vi "PulseParseSequence.vi"(0 "String":string) -> (1 "Step invarient?":bool, 2 "pulses cluster":T1)   [LabVIEW 2017]
panel:
  out "Camera String":string
  out "Sequences cluster":T2
  out "RF String":string
  out "Main Pulses String":string
  out "Synths String":string
  out "Pars String":string
  out "Aux Pulses String":string
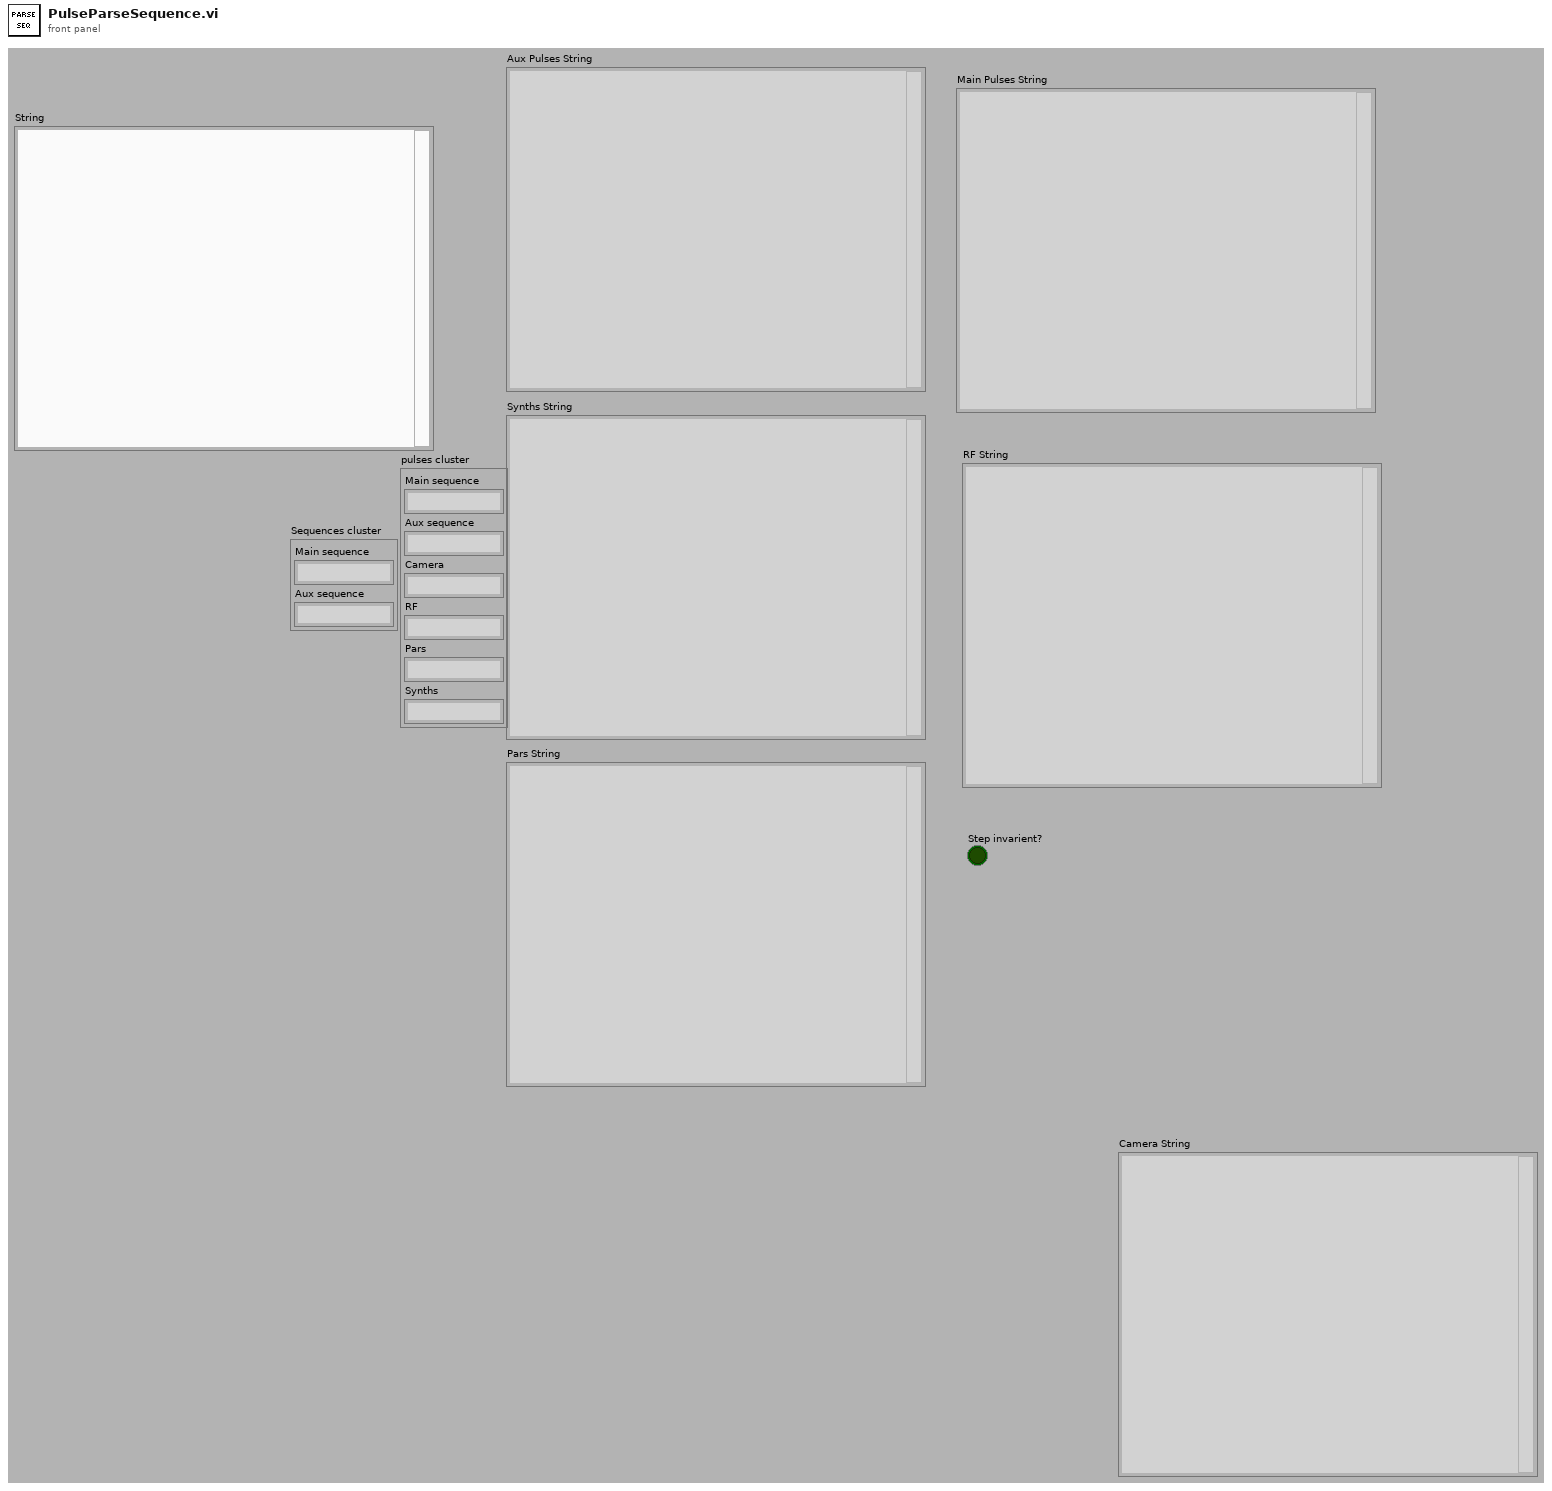
[diagram p1: front panel]
types:
  T1 = cluster{"Main sequence":string, "Aux sequence":string, "Camera":string, "RF":string, "Pars":string, "Synths":string}
  T2 = cluster{"Main sequence":string, "Aux sequence":string}
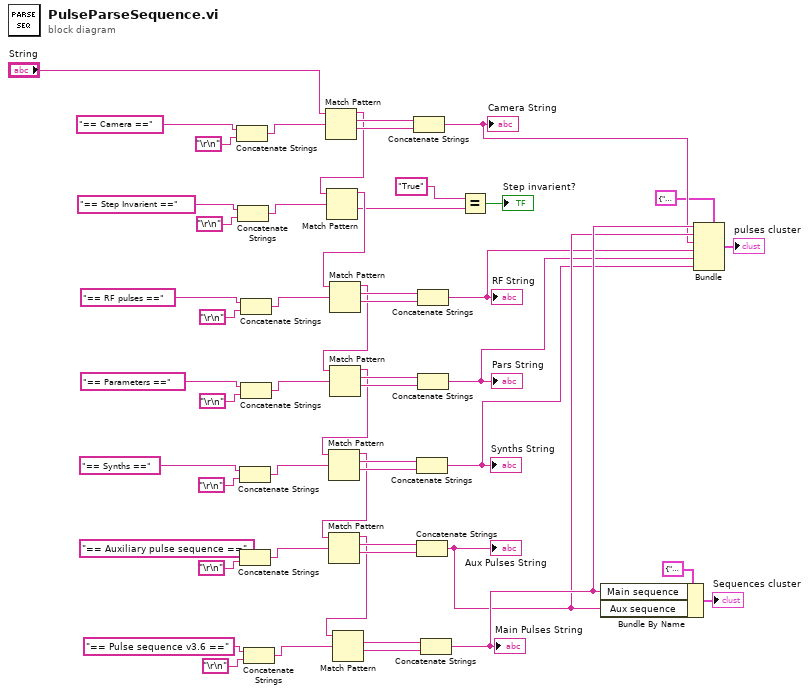
[diagram p0: block diagram]
diagram:
  n1 = Concatenate Strings("== Camera ==", "\r\n") -> (w15:string)
  n2 = Concatenate Strings("== Step Invarient ==", "\r\n") -> (w22:string)
  n3 = Concatenate Strings("== Synths ==", "\r\n") -> (w43:string)
  n4 = Concatenate Strings("== Auxiliary pulse sequence ==", "\r\n") -> (w53:string)
  n5 = Concatenate Strings("== RF pulses ==", "\r\n") -> (w30:string)
  n6 = Concatenate Strings("== Parameters ==", "\r\n") -> (w48:string)
  n7 = Concatenate Strings("== Pulse sequence v3.6 ==", "\r\n") -> (w36:string)
  n8 = Match Pattern(string="String", regular expression=w15) -> (before substring=w10:string, match substring=w11:string, after substring=w12:string)  [unwired: 1 in, 1 out]
  n9 = Match Pattern(string=w10, regular expression=w22) -> (before substring=w19:string, after substring=w18:string)  [unwired: 1 in, 2 out]
  n10 = Match Pattern(string=w19, regular expression=w30) -> (before substring=w25:string, match substring=w26:string, after substring=w27:string)  [unwired: 1 in, 1 out]
  n11 = Match Pattern(string=w25, regular expression=w48) -> (before substring=w38:string, match substring=w44:string, after substring=w45:string)  [unwired: 1 in, 1 out]
  n12 = Match Pattern(string=w38, regular expression=w43) -> (before substring=w37:string, match substring=w39:string, after substring=w40:string)  [unwired: 1 in, 1 out]
  n13 = Match Pattern(string=w37, regular expression=w53) -> (before substring=w31:string, match substring=w49:string, after substring=w50:string)  [unwired: 1 in, 1 out]
  n14 = Match Pattern(string=w31, regular expression=w36) -> (match substring=w32:string, after substring=w33:string)  [unwired: 1 in, 2 out]
  n15 = Concatenate Strings(w11, w12) -> (w6:string)
  "Camera String" <- w6
  n16 = Concatenate Strings(w39, w40) -> (w3:string)
  "Synths String" <- w3
  n17 = Concatenate Strings(w49, w50) -> (w7:string)
  "Aux Pulses String" <- w7
  n18 = Concatenate Strings(w26, w27) -> (w5:string)
  "RF String" <- w5
  n19 = Concatenate Strings(w44, w45) -> (w4:string)
  "Pars String" <- w4
  n20 = Concatenate Strings(w32, w33) -> (w8:string)
  "Main Pulses String" <- w8
  n21 = Equal?(x="True", y=w18) -> (x = y?=→"Step invarient?":bool)
  n22 = Bundle By Name(cluster=T2 {"Main sequence"="", "Aux sequence"=""} ("Sequences cluster"), "Main sequence"=w8, "Aux sequence"=w7) -> (→"Sequences cluster":T2)
  n23 = Bundle(cluster=T1 {"Main sequence"="", "Aux sequence"="", "Camera"="", "RF"="", "Pars"="", "Synths"=""} ("output cluster"), "Main sequence"=w8, "Aux sequence"=w7, "Camera"=w6, "RF"=w5, "Pars"=w4, "Synths"=w3) -> (→"pulses cluster":T1)
